vi "traj_generator_test.vi"() -> ()   [LabVIEW 2014]
panel:
  in  "stop":bool
  in  "p_f":dbl
  in  "Trigger":bool
  out "Waveform Chart":cluster{"p":dbl, "v":dbl, "a":dbl}(graph)
  # "<--- Taerget"
  # "<--- Triggered by rising edge"
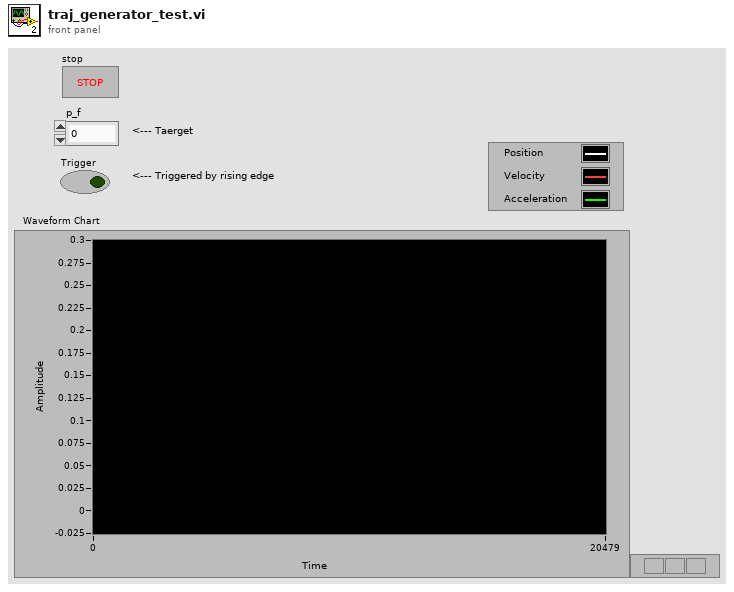
[diagram p1: front panel]
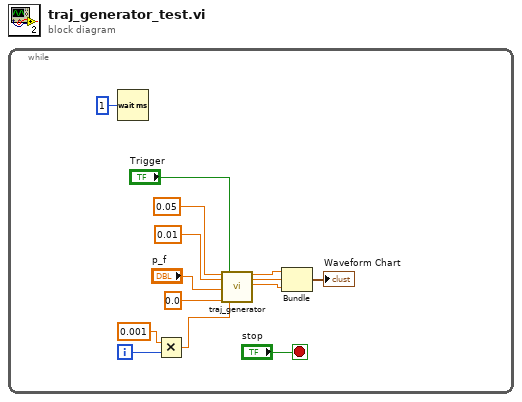
[diagram p0: block diagram]
diagram:
  n1 = while {
    i -> [w14]
    stop <- "stop" stop-if-true
    n2 = Wait (ms)(milliseconds to wait=u32 1) -> ()  [unwired: 1 out]
    n3 = Multiply(x=0.001, y=w14) -> (x*y=w11:dbl)
    n4 = call "traj_generator.vi"("v_max"=0.05, "a_max"=0.01, "p_f"="p_f", "v_f"=0.0 ("p_i"), "trigger"="Trigger", "t"=w11) -> ("p"=w8:dbl, "v"=w7:dbl, "a"=w1:dbl)  [unwired: 11 in]
    n5 = Bundle("p"=w8, "v"=w7, "a"=w1) -> (→"Waveform Chart":cluster{"p":dbl, "v":dbl, "a":dbl})  [unwired: 1 in]
  }
